vi "GenerateOverriddenSystemDefinitionFromExplicitOverrides.vi"(8 "error in (no error)":errorcluster, 9 "Targets Configuration":T1, 10 "overrides":T3[](array[typedef]), 11 "absolute system definition file":path) -> (0 "error out":errorcluster, 1 "Temporary File?":bool, 3 "absolute overridden system definition file":path)   [LabVIEW 2027, in "VeriStandTestUtilities.lvlib"]
uses:
  VeriStandTestUtilities.lvlib
  ConfigOverrideItem.ctl
  TargetsConfiguration.ctl
  TargetPlatform.ctl
  C:/NetCoreDLL/NationalInstruments.VeriStand.SystemDefinitionAPI.dll
  NetCoreDLL/NationalInstruments.VeriStand.SystemDefinitionAPI.dll
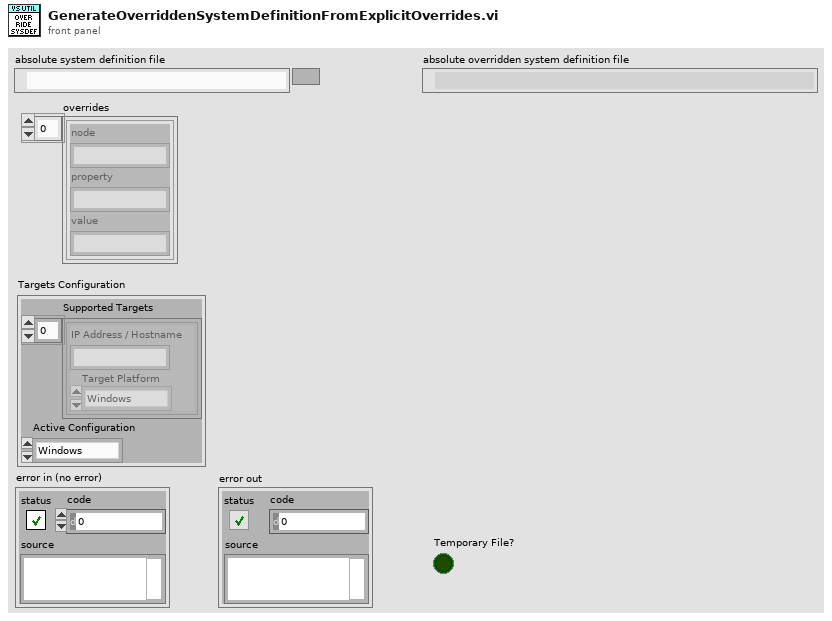
[diagram p1: front panel]
types:
  T1 = typedef "VeriStandTestUtilities.lvlib/TargetsConfiguration.ctl" = cluster{"Supported Targets":cluster{"IP Address / Hostname":string, "Target Platform":T2}[], "Active Configuration":T2}
  T2 = typedef "VeriStandTestUtilities.lvlib/TargetPlatform.ctl" = enum16{"Windows", "Linux64CRIO", "Linux64PXI", "LinuxARM", "PharLap"}
  T3 = typedef "VeriStandTestUtilities.lvlib/ConfigOverrideItem.ctl" = cluster{"node":string, "property":string, "value":string}
  T4 = cluster{"IP Address / Hostname":string, "Target Platform":T2}[]
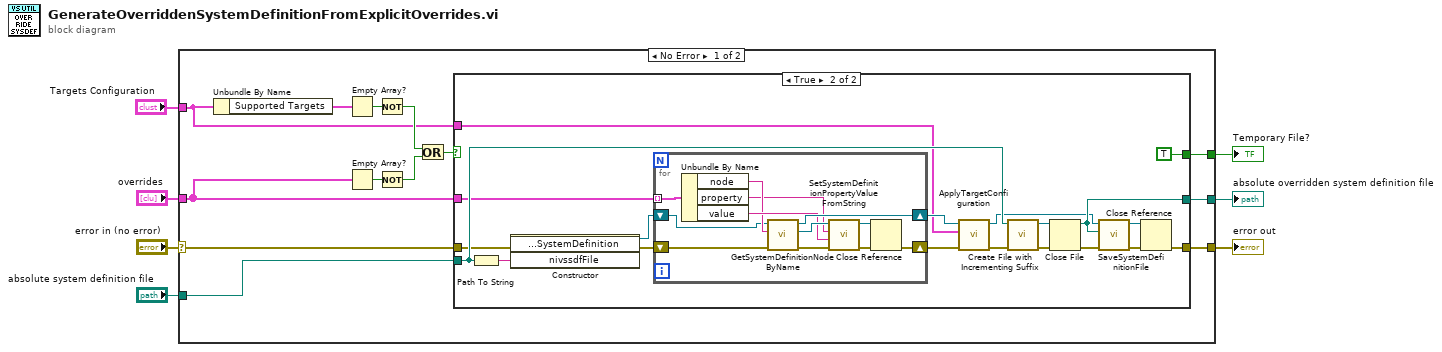
[diagram p0: block diagram]
diagram:
  n1 = case shown="No Error" "error in (no error)" {
    selector: "error in (no error)" -> [w20 w55]
    tunnel: "absolute system definition file" -> [w19 w54]
    tunnel: [w18 w55] -> w5
    tunnel: [w17 w54] -> w4
    tunnel: [w16 _] -> w3
    tunnel: "overrides" -> [w15 _]
    tunnel: "Targets Configuration" -> [w8 _]
    frame No Error {
      n2 = Unbundle By Name(w8) -> ("Supported Targets"=w13:T4)
      n3 = Empty Array?(array=w13) -> (empty?=w14:bool)
      n4 = Empty Array?(array=w15) -> (empty?=w12:bool)
      n5 = Not(x=w14) -> (.not. x?=w10:bool)
      n6 = Not(x=w12) -> (.not. x?=w11:bool)
      n7 = Or(x=w10, y=w11) -> (x .or. y?=w9:bool)
      n8 = case shown="True" w9 {
        tunnel: w20 -> [w21 w28]
        tunnel: w19 -> [w22 w35]
        tunnel: [w21 w38] -> w18
        tunnel: [w22 w31] -> w17
        tunnel: [_ TRUE ("Temporary File?")] -> w16
        tunnel: w15 -> [_ w29]
        tunnel: w8 -> [_ w23]
        frame False {
        }
        frame True {
          n9 = Path To String(path=w35) -> (string=w39:string)
          n10 = constructor class="SystemDefinition"(error in=w28, "nivssdfFile"=w39) -> (reference out=w41:refnum<k39>, error out=w40:errorcluster)  [unwired: 2 in, 2 out]
          n11 = for {
            shift-right: [w48] -> w24
            shift-left: w41 -> [w42]
            shift-right: [w49] -> w26
            shift-left: w40 -> [w45]
            tunnel: w29 -> [w47] mode=indexing
            n12 = Unbundle By Name(w47) -> ("node"=w44:string, "property"=w43:string, "value"=w46:string)
            n13 = call "GetSystemDefinitionNodeByName.vi"("error in (no error)"=w45, "nodepath"=w44, "NationalInstruments.VeriStand.SystemDefinitionAPI.SystemDefinition"=w42) -> ("error out"=w52:errorcluster, "NationalInstruments.VeriStand.SystemStorage.BaseNodeType"=w53:refnum<k39>, "NationalInstruments.VeriStand.SystemDefinitionAPI.SystemDefinition"=w48:refnum<k39>)  [unwired: 6 in]
            n14 = call "SetSystemDefinitionPropertyValueFromString.vi"("error in (no error)"=w52, "value"=w46, "property name"=w43, "NationalInstruments.VeriStand.SystemStorage.BaseNodeType"=w53) -> ("error out"=w50:errorcluster, "NationalInstruments.VeriStand.SystemStorage.BaseNodeType"=w51:refnum<k39>)  [unwired: 6 in]
            n15 = Close Reference(reference=w51, error in (no error)=w50) -> (error out=w49:errorcluster)
          }
          n16 = call "ApplyTargetConfiguration.vi"("error in (no error)"=w26, "Targets Configuration"=w23, "NationalInstruments.VeriStand.SystemDefinitionAPI.SystemDefinition"=w24) -> ("error out"=w27:errorcluster, "NationalInstruments.VeriStand.SystemDefinitionAPI.SystemDefinition"=w25:refnum<k39>)  [unwired: 7 in]
          n17 = call <vilib>:"Create File with Incrementing Suffix.vi"("error in (no error)"=w27, "file path"=w35) -> ("error out"=w34:errorcluster, "refnum out"=w32:refnum<file>)  [unwired: 7 in, 1 out]
          n18 = Close File(refnum=w32, error in=w34) -> (path=w31:path, error out=w33:errorcluster)
          n19 = call "SaveSystemDefinitionFile.vi"("error in (no error)"=w33, "System Definition File in"=w31, "NationalInstruments.VeriStand.SystemDefinitionAPI.SystemDefinition"=w25) -> ("error out"=w37:errorcluster, "NationalInstruments.VeriStand.SystemDefinitionAPI.SystemDefinition"=w36:refnum<k39>)  [unwired: 7 in]
          n20 = Close Reference(reference=w36, error in (no error)=w37) -> (error out=w38:errorcluster)
        }
      }
    }
    frame Error {
    }
  }
  "error out" <- w5
  "absolute overridden system definition file" <- w4
  "Temporary File?" <- w3
